vi "Release Control Cluster.vi"(11 "output cluster":T1) -> ()   [LabVIEW 2019, in "Controller.lvclass"]
uses:
  Controller.lvclass
  Controllers.ctl
  I-O/I-O.lvclass
  Dispenser/Dispenser.lvclass
  C:/Program Files (x86)/Aerotech/A3200/LabVIEW/2010/Bin/Aerotech.A3200.dll
  Program Files (x86)/Aerotech/A3200/LabVIEW/2010/Bin/Aerotech.A3200.dll
  Motion/A3200/A3200.lvclass
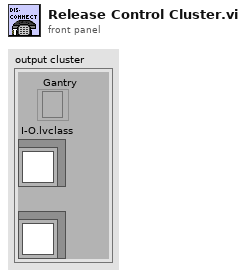
[diagram p1: front panel]
types:
  T1 = typedef "Controller.lvclass/Controllers.ctl" = cluster{"I-O.lvclass":refnum<class "I-O.lvclass">, "Dispenser.lvclass":refnum<class "Dispenser.lvclass">, "Gantry":refnum<k24>}
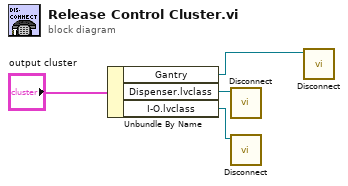
[diagram p0: block diagram]
diagram:
  n1 = Unbundle By Name("output cluster") -> ("Gantry"=w3:refnum<k24>, "Dispenser.lvclass"=w1:refnum<class "Dispenser.lvclass">, "I-O.lvclass"=w2:refnum<class "I-O.lvclass">)
  n2 = call-dynamic "Disconnect.vi"("Controller in"=w1) -> ()  [unwired: 9 in, 1 out]
  n3 = call-dynamic "Disconnect.vi"("I-O in"=w2) -> ()  [unwired: 9 in, 1 out]
  n4 = call "Disconnect.vi"("Gantry In"=w3) -> ()  [unwired: 9 in, 1 out]
